vi "HEWH Build Heating Source Array SUo.vi"(4 "Take Sample at 5 Min":bool, 6 "Qr (T), SU0 (F)":bool, 7 "5 Minute Subset Index Adder":i32, 8 "error in (no error)":errorcluster, 9 "Elapsed Time (sec)":dbl[](array[numeric]), 10 "TC Tree Average":dbl[](array[numeric]), 11 "UEF Calculated Values":T1 {"Data Indexes"."15 sec after Draw Index" format="%#.2f"; "Data Indexes"."15 sec after Draw Timestamp" format="%#.2f"; "Data Indexes"."Test Start Timestamp" format="%.2f"; "Data Indexes"."Test End Timestamp" format="%.2f"; "Data Indexes"."T0 Timestamp" format="%.2f"; "Data Indexes"."Tsf Timestamp" format="%.2f"; "Data Indexes"."Tsu0 Timestamp" format="%.2f"; "Data Indexes"."Tmax1 Timestamp" format="%.2f"; "Data Indexes"."Draw Index Timestamp" format="%#.2f"; "Data Indexes"."Non-Draw Timestamp" format="%#.2f"; "Data Indexes"."Heating Timestamp" format="%#.2f"; "Data Indexes"."Start Energy (BTU-Gas)" format="%.6f"; "Data Indexes"."Start Watt Hours" format="%.6f"; "Static Data"."V - Volume of Wh (True)" format="%.5f"; "Static Data"."T-Ambinet Nominal (°F)" format="%.5f"; "Static Data"."T-Inlet Setpoint (°F)" format="%.5f"; "Static Data"."T-Wh Setpoint (°F)" format="%.5f"; "Sampled Data"."Qe (Wh)" format="%.5f"; "Sampled Data"."Tau stby2 (hr)" format="%.5f"; "Sampled Data"."Tastby2 (°F)" format="%.5f"; "Sampled Data"."Qf (BTU)" format="%.5f"; "Sampled Data"."Qe (BTU)" format="%.5f"; "Sampled Data"."Tmax1 (°F)" format="%.5f"; "Sampled Data"."T0 (°F)" format="%.5f"; "Sampled Data"."Qr (BTU)" format="%.5f"; "Sampled Data"."T 24(°F)" format="%.5f"; "Sampled Data"."T astby(°F)" format="%.5f"; "Sampled Data"."T tstby(°F)" format="%.5f"; "Sampled Data"."T su0(°F)" format="%.5f"; "Sampled Data"."T suf(°F)" format="%.5f"; "Sampled Data"."Tau stby_1 (hr)" format="%.5f"; "Sampled Data"."Qsuf (BTU)" format="%.5f"; "Sampled Data"."Qsu0 (BTU)" format="%.5f"; "Calculated Values"."Draw Bonus Volume (gal)" format="%.6f"; "Calculated Values"."Adjustment Factor" format="%.6f"; "Calculated Values"."T*avg_del(n-1)" format="%.6f"; "Calculated Values"."T*min(n-1)" format="%.6f"; "Calculated Values"."T*avg_del(n)" format="%.6f"; "Calculated Values"."Vn" format="%.6f"; "Calculated Values"."Qdm (BTU)" format="%.6f"; "Calculated Values"."QHWD (BTU)" format="%.6f"; "Calculated Values"."QHW (BTU)" format="%.6f"; "Calculated Values"."UEF" format="%.6f"; "Calculated Values"."QHW67 (BTU)" format="%.6f"; "Calculated Values"."Qda (BTU)" format="%.6f"; "Calculated Values"."Qd (BTU)" format="%.6f"; "Calculated Values"."Q (BTU)" format="%.6f"; "Calculated Values"."UA (BTU/(hr*F))" format="%.6f"; "Calculated Values"."Qhr (BTU/hr)" format="%.6f"; "Calculated Values"."Qstby (BTU)" format="%.6f"; "Calculated Values"."nu_r" format="%.6f"; "Calculated Values"."CpUEF (BTU/(lb*F))" format="%.6f"; "Calculated Values"."rho_nu (lb/gal)" format="%.6f"; "Calculated Values"."V1- Vol (Gal)" format="%.6f"; "Calculated Values"."M cluster mass removed (lb)" format="%.6f"; "Calculated Values"."Cp theoretical (BTU/(lbm °F))" format="%.6f"; "Calculated Values"."Tin1 - Mean Inlet 1st Cluster (°F)" format="%.6f"; "Calculated Values"."Tdel1-Mean Outlet 1st Cluster(°F)" format="%.6f"; "Calculated Values"."Cp 24 (BTU/(lb*F))" format="%.6f"; "Calculated Values"."Cp standby (BTU/(lb*F))" format="%.6f"; "Calculated Values"."Cp2 (BTU/(lb*F))" format="%.6f"; "Calculated Values"."Cp1 (BTU/(lb*F))" format="%.6f"; "Calculated Values"."rho 24 (lb/gal)" format="%.6f"; "Calculated Values"."rho standby (lb/gal)" format="%.6f"; "Calculated Values"."rho 2 (lb/gal)" format="%.6f"; "Calculated Values"."Density of cold water All (lbm/gal)" format="%#.3g"; "Calculated Values"."CpHW (BTU/(lbm °F))" format="%#.3g"; "Calculated Values"."Density of hot water All (lbm/gal)" format="%#.3g"; "Calculated Values"."Mass of water All (lbm)" format="%#.3f"}) -> (0 "error out":errorcluster, 1 "Subset Index":i32, 2 "max index(es)":i32, 3 "max value":dbl, 5 "New End Index":i32)   [LabVIEW 2023]
uses:
  Type Definitions/UEF Constants.ctl
  Type Definitions/HEWH Draw Stats.ctl
  Type Definitions/HEWH FHR Draw Type.ctl
  Type Definitions/FHR Bins.ctl
  Type Definitions/HEWH Meter Type.ctl
panel:
  out "subarray":dbl[](array[numeric])
  # "FHR"
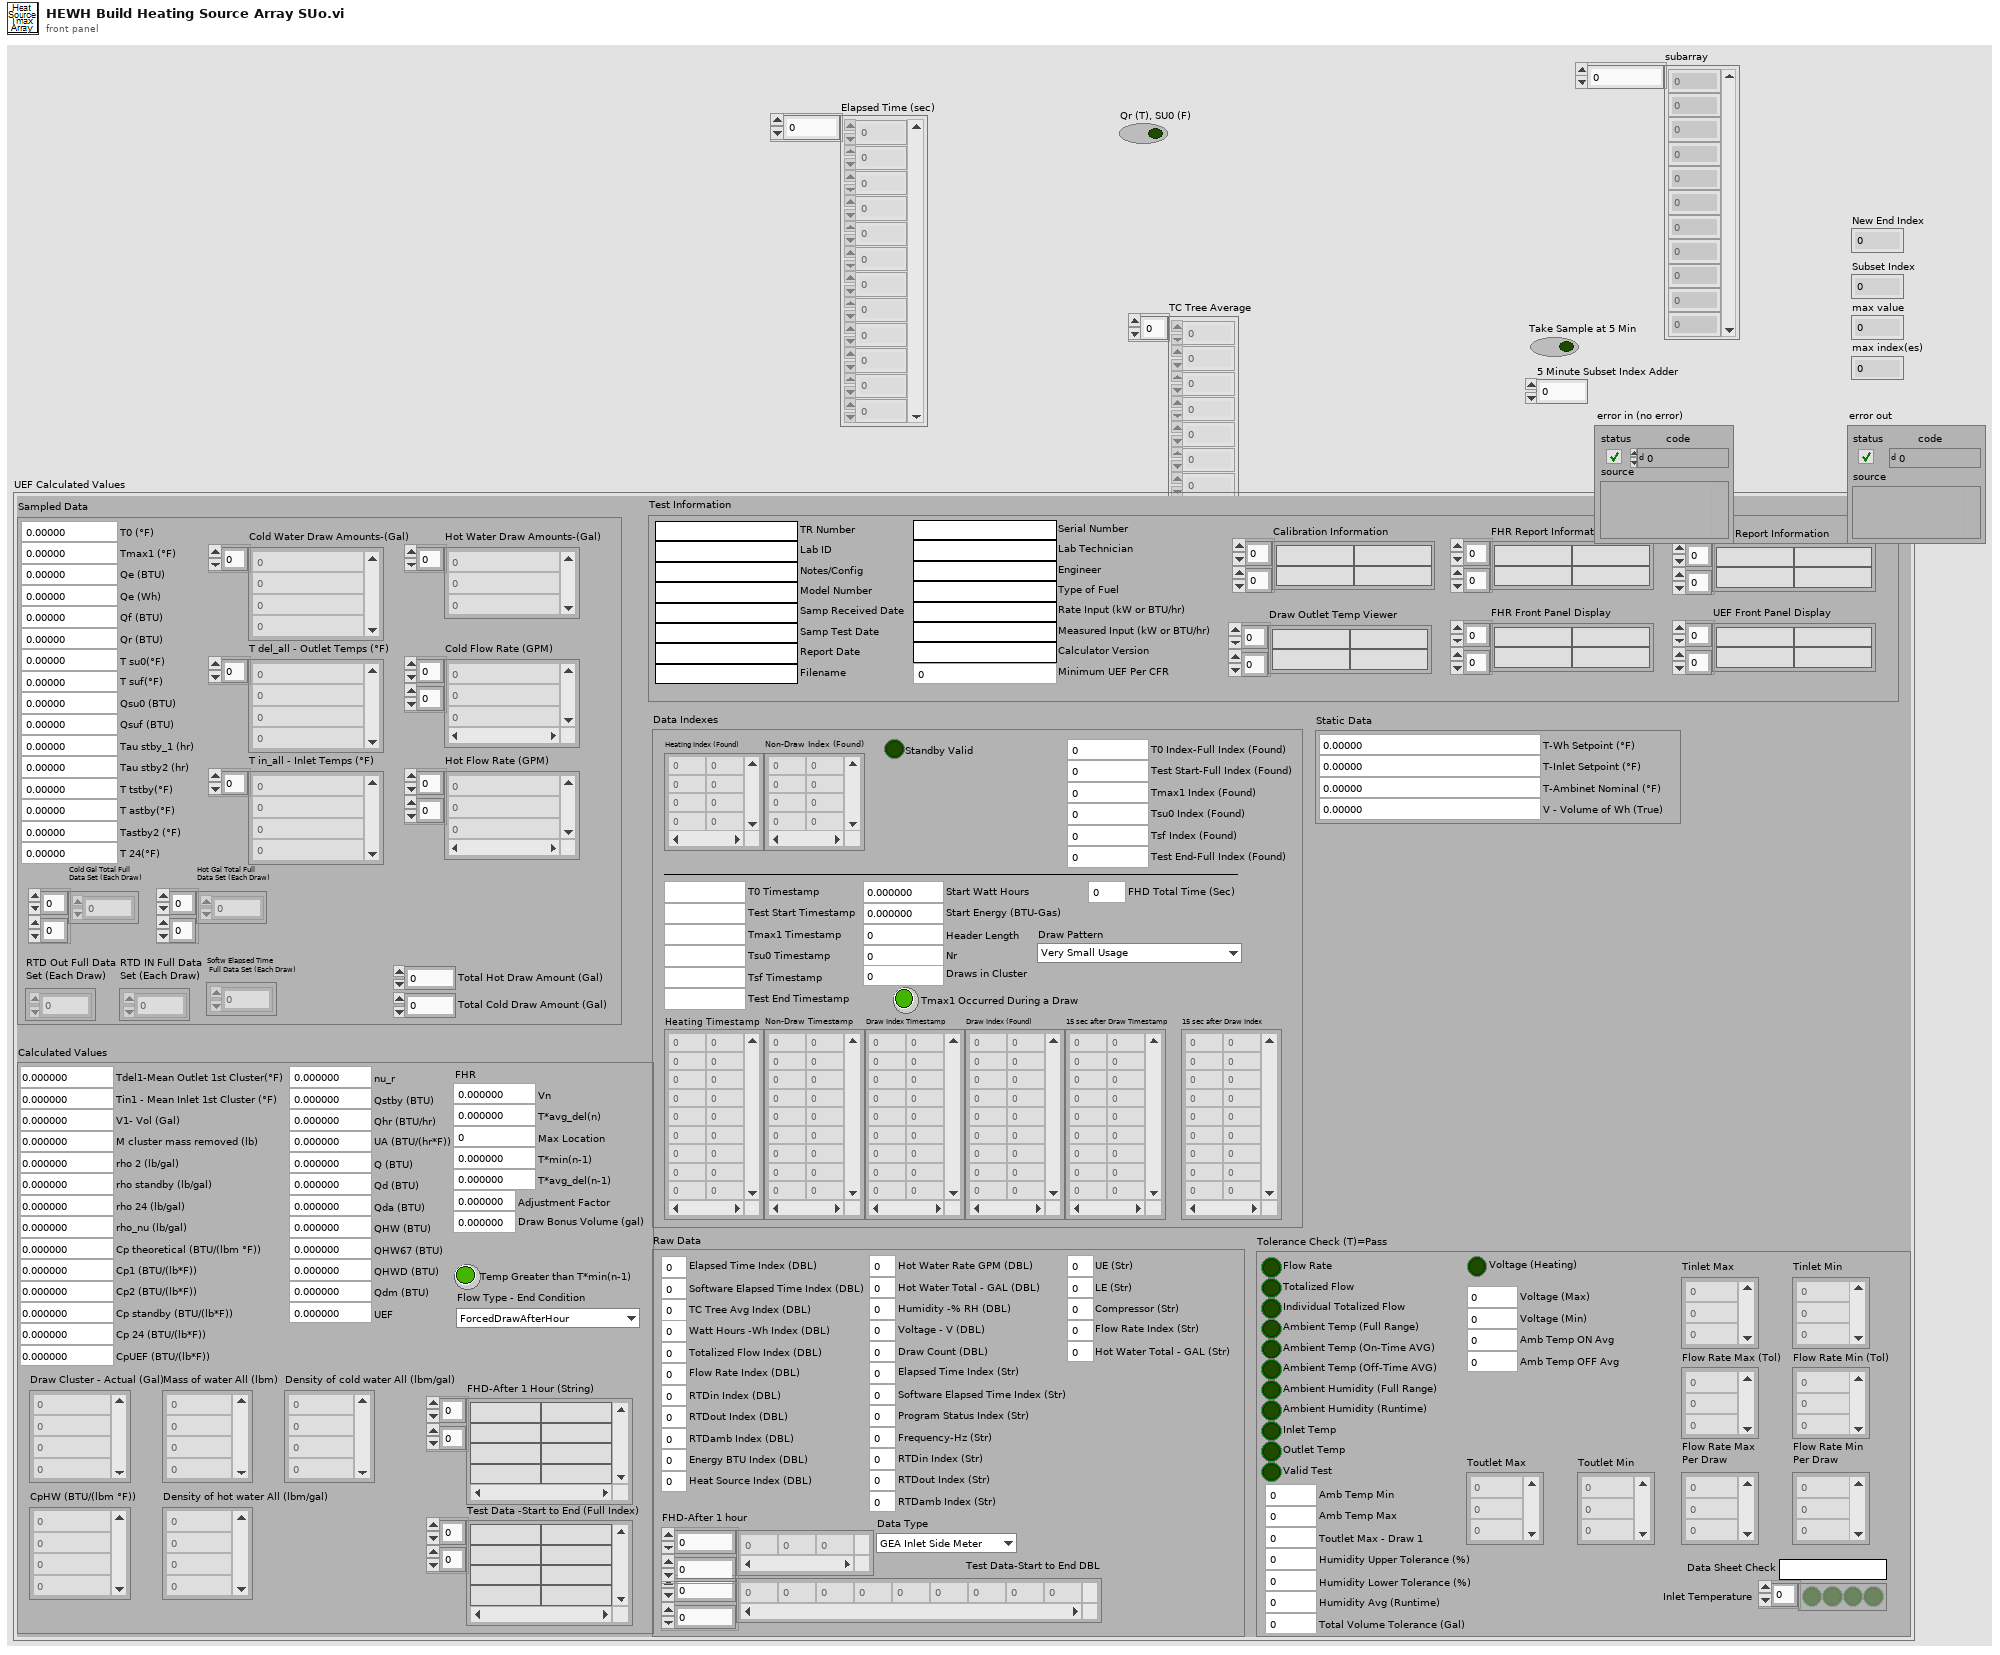
[diagram p1: front panel]
types:
  T1 = typedef "UEF Constants.ctl" = cluster{"Calculated Values":T2, "Sampled Data":cluster{"Cold Water Draw Amounts-(Gal)":dbl[], "T del_all - Outlet Temps (°F)":dbl[], "T in_all - Inlet Temps (°F)":dbl[], "Qsu0 (BTU)":dbl, "Qsuf (BTU)":dbl, "Tau stby_1 (hr)":dbl, "T suf(°F)":dbl, "T su0(°F)":dbl, "T tstby(°F)":dbl, "T astby(°F)":dbl, "T 24(°F)":dbl, "Qr (BTU)":dbl, "T0 (°F)":dbl, "Tmax1 (°F)":dbl, "Qe (BTU)":dbl, "Qf (BTU)":dbl, "Tastby2 (°F)":dbl, "RTD Out Full Data\nSet (Each Draw)":dbl[][], "RTD IN Full Data\nSet (Each Draw)":dbl[][], "Tau stby2 (hr)":dbl, "Hot Water Draw Amounts-(Gal)":dbl[], "Cold Flow Rate (GPM)":dbl[][], "Hot Flow Rate (GPM)":dbl[][], "Softw Elapsed Time\n Full Data Set (Each Draw)":dbl[][], "Cold Gal Total Full\nData Set (Each Draw)":dbl[][], "Total Hot Draw Amount (Gal) ":dbl, "Total Cold Draw Amount (Gal)":dbl, "Qe (Wh)":dbl, "Hot Gal Total Full\nData Set (Each Draw)":dbl[][]}, "Static Data":cluster{"T-Wh Setpoint (°F)":dbl, "T-Inlet Setpoint (°F)":dbl, "T-Ambinet Nominal (°F)":dbl, "V - Volume of Wh (True)":dbl}, "Data Indexes":cluster{"Test Start-Full Index (Found)":i32, "Header Length":i32, "Draw Index (Found)":i32[][], "Nr":i32, "Start Watt Hours":dbl, "Tsu0 Index (Found)":i32, "Tsf Index (Found)":i32, "Start Energy (BTU-Gas)":dbl, "Draws in Cluster":i32, "T0 Index-Full Index (Found)":i32, "Non-Draw Index (Found)":i32[][], "Tmax1 Index (Found)":i32, "Test End-Full Index (Found)":i32, "Heating Index (Found)":i32[][], "Heating Timestamp":dbl[][], "Non-Draw Timestamp":dbl[][], "Draw Index Timestamp":dbl[][], "Tmax1 Timestamp":dbl, "Tsu0 Timestamp":dbl, "Tsf Timestamp":dbl, "T0 Timestamp":dbl, "Test End Timestamp":dbl, "Test Start Timestamp":dbl, "15 sec after Draw Timestamp":dbl[][], "15 sec after Draw Index":dbl[][], "Tmax1 Occurred During a Draw":bool, "FHD Total Time (Sec)":dbl, "Draw Pattern":T4, "Standby Valid":bool}, "Raw Data":cluster{"Elapsed Time Index (DBL)":i32, "Software Elapsed Time Index (DBL)":i32, "TC Tree Avg Index (DBL)":i32, "Watt Hours -Wh Index (DBL)":i32, "Energy BTU Index (DBL)":i32, "Totalized Flow Index (DBL)":i32, "Flow Rate Index (DBL)":i32, "Program Status Index (Str)":i32, "RTDin Index (DBL)":i32, "RTDout Index (DBL)":i32, "RTDamb Index (DBL)":i32, "Test Data-Start to End DBL":dbl[][], "Data Type":T5, "Heat Source Index (DBL)":i32, "Hot Water Rate GPM (DBL)":i32, "Hot Water Total - GAL (DBL)":i32, "FHD-After 1 hour":dbl[][], "Humidity -% RH (DBL)":i32, "Voltage - V (DBL)":i32, "Draw Count (DBL)":i32, "Elapsed Time Index (Str)":i32, "Software Elapsed Time Index (Str)":i32, "Frequency-Hz (Str)":i32, "RTDin Index (Str)":i32, "RTDout Index (Str)":i32, "RTDamb Index (Str)":i32, "UE (Str)":i32, "LE (Str)":i32, "Compressor (Str)":i32, "Flow Rate Index (Str)":i32, "Hot Water Total - GAL (Str)":i32}, "Tolerance Check (T)=Pass":cluster{"Flow Rate":bool, "Totalized Flow":bool, "Ambient Temp (Full Range)":bool, "Ambient Humidity (Full Range)":bool, "Inlet Temp":bool, "Outlet Temp":bool, "Valid Test":bool, "Individual Totalized Flow":bool, "Data Sheet Check":string, "Inlet Temperature":bool[], "Tinlet Max":dbl[], "Tinlet Min":dbl[], "Flow Rate Max (Tol)":dbl[], "Flow Rate Min (Tol)":dbl[], "Amb Temp Max":dbl, "Amb Temp Min":dbl, "Toutlet Max - Draw 1":dbl, "Humidity Upper Tolerance (%)":dbl, "Total Volume Tolerance (Gal)":dbl, "Humidity Lower Tolerance (%)":dbl, "Flow Rate Max\nPer Draw":dbl[], "Flow Rate Min\nPer Draw":dbl[], "Ambient Humidity (Runtime)":bool, "Humidity Avg (Runtime)":dbl, "Ambient Temp (On-Time AVG)":bool, "Ambient Temp (Off-Time AVG)":bool, "Amb Temp OFF Avg":dbl, "Amb Temp ON Avg":dbl, "Voltage (Heating)":bool, "Voltage (Min)":dbl, "Voltage (Max)":dbl, "Toutlet Max":dbl[], "Toutlet Min":dbl[]}, "Test Information":cluster{"TR Number":string, "Lab ID":string, "Notes/Config":string, "Model Number":string, "Serial Number":string, "Lab Technician":string, "Engineer":string, "Type of Fuel":string, "Samp Received Date":string, "Samp Test Date":string, "Report Date":string, "Rate Input (kW or BTU/hr)":string, "Measured Input (kW or BTU/hr)":string, "Filename":string, "Calibration Information":string[][], "Calculator Version":string, "Minimum UEF Per CFR":dbl, "UEF Report Information":string[][], "FHR Report Information":string[][], "FHR Front Panel Display":string[][], "UEF Front Panel Display":string[][], "Draw Outlet Temp Viewer":string[][]}}
  T2 = typedef "HEWH Draw Stats.ctl" = cluster{"Draw Cluster - Actual (Gal)":dbl[], "Mass of water All (lbm)":dbl[], "Density of hot water All (lbm/gal)":dbl[], "CpHW (BTU/(lbm °F))":dbl[], "rho 2 (lb/gal)":dbl, "rho standby (lb/gal)":dbl, "rho 24 (lb/gal)":dbl, "Cp1 (BTU/(lb*F))":dbl, "Cp2 (BTU/(lb*F))":dbl, "Cp standby (BTU/(lb*F))":dbl, "Cp 24 (BTU/(lb*F))":dbl, "nu_r":dbl, "Qstby (BTU)":dbl, "Qhr (BTU/hr)":dbl, "UA (BTU/(hr*F))":dbl, "Q (BTU)":dbl, "Qd (BTU)":dbl, "Qda (BTU)":dbl, "QHW67 (BTU)":dbl, "UEF":dbl, "Tdel1-Mean Outlet 1st Cluster(°F)":dbl, "Tin1 - Mean Inlet 1st Cluster (°F)":dbl, "Cp theoretical (BTU/(lbm °F))":dbl, "M cluster mass removed (lb)":dbl, "V1- Vol (Gal)":dbl, "Test Data -Start to End (Full Index)":string[][], "rho_nu (lb/gal)":dbl, "Density of cold water All (lbm/gal)":dbl[], "CpUEF (BTU/(lb*F))":dbl, "QHW (BTU)":dbl, "QHWD (BTU)":dbl, "Qdm (BTU)":dbl, "FHD-After 1 Hour (String)":string[][], "Vn":dbl, "T*avg_del(n)":dbl, "Max Location":i32, "T*min(n-1)":dbl, "T*avg_del(n-1)":dbl, "Temp Greater than T*min(n-1)":bool, "Adjustment Factor":dbl, "Draw Bonus Volume (gal)":dbl, "Flow Type - End Condition":T3}
  T3 = typedef "HEWH FHR Draw Type.ctl" = enum16{"ForcedDrawAfterHour", "HeatingCutoffBeforeHour"}
  T4 = typedef "FHR Bins.ctl" = enum16{"Very Small Usage", "Low Usage", "Medium Usage", "High Usage", "Undefined"}
  T5 = typedef "HEWH Meter Type.ctl" = enum16{"GEA Inlet Side Meter", "GEA Outlet Side Meter", "CSA Inlet Side Meter"}
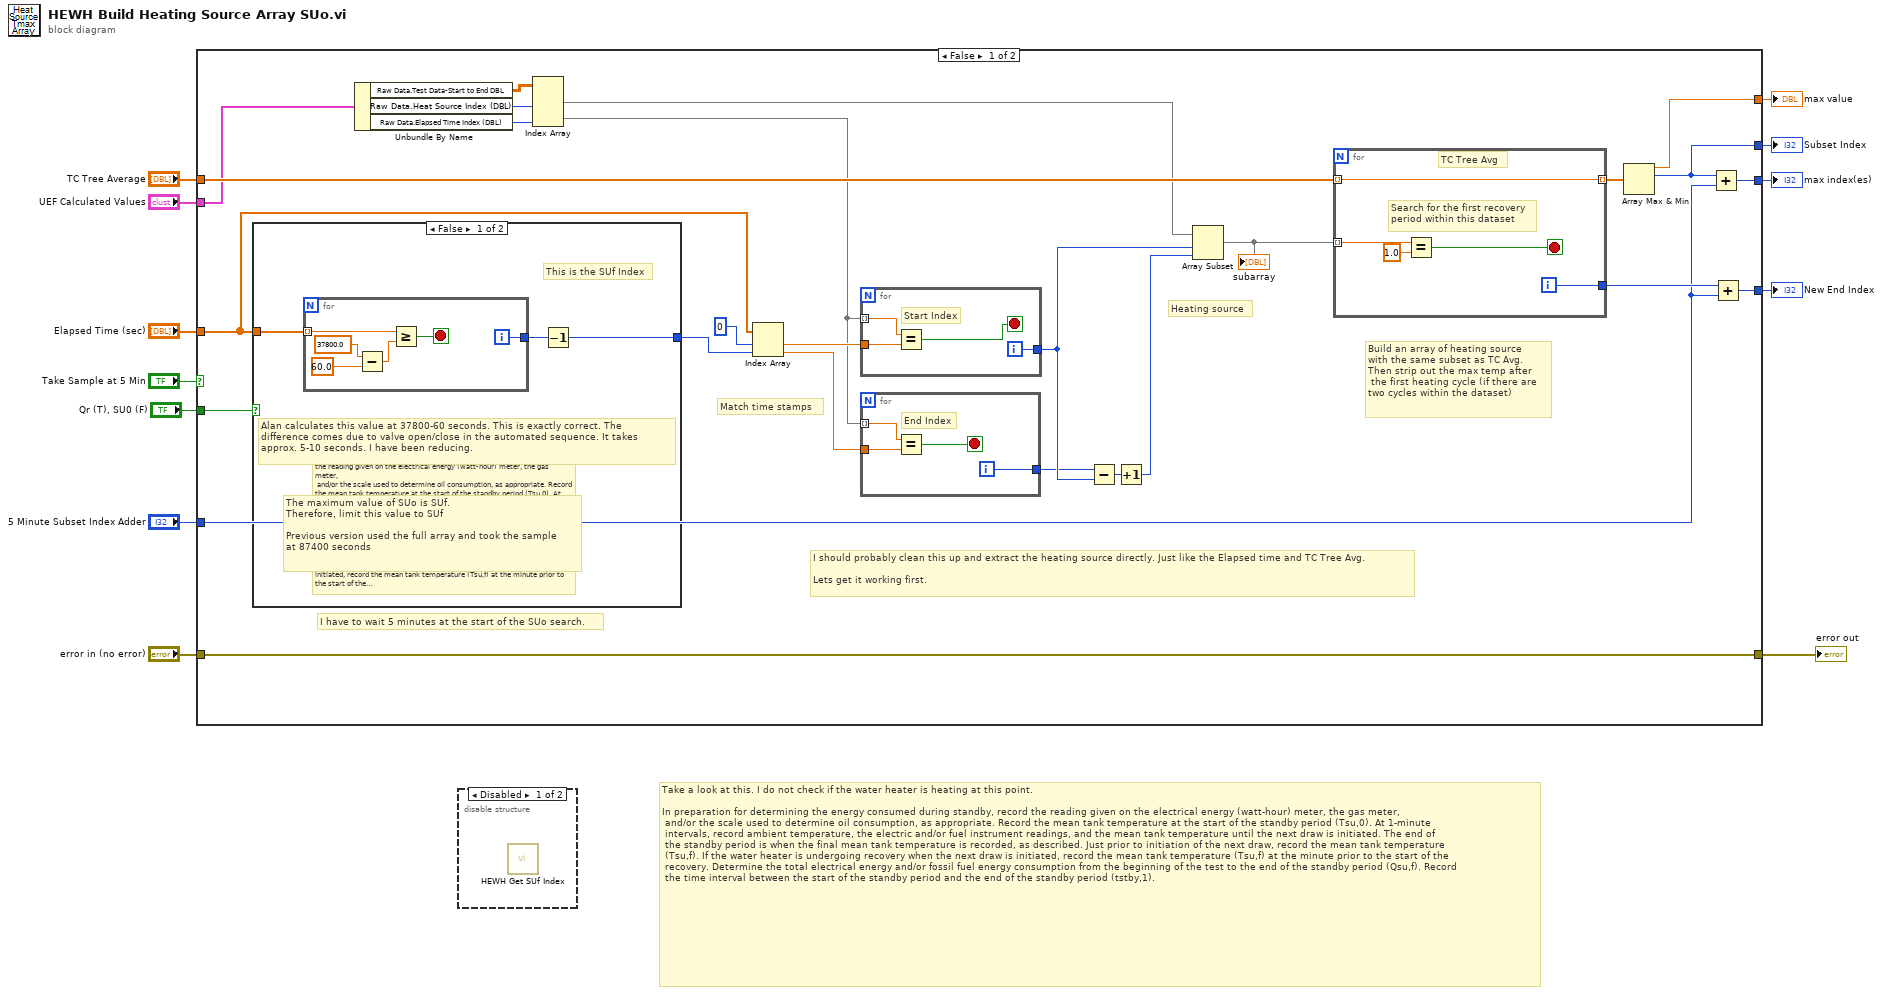
[diagram p0: block diagram]
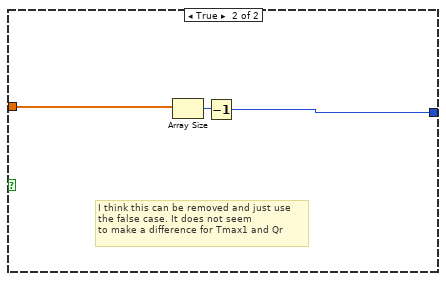
[diagram p3: hidden frame]
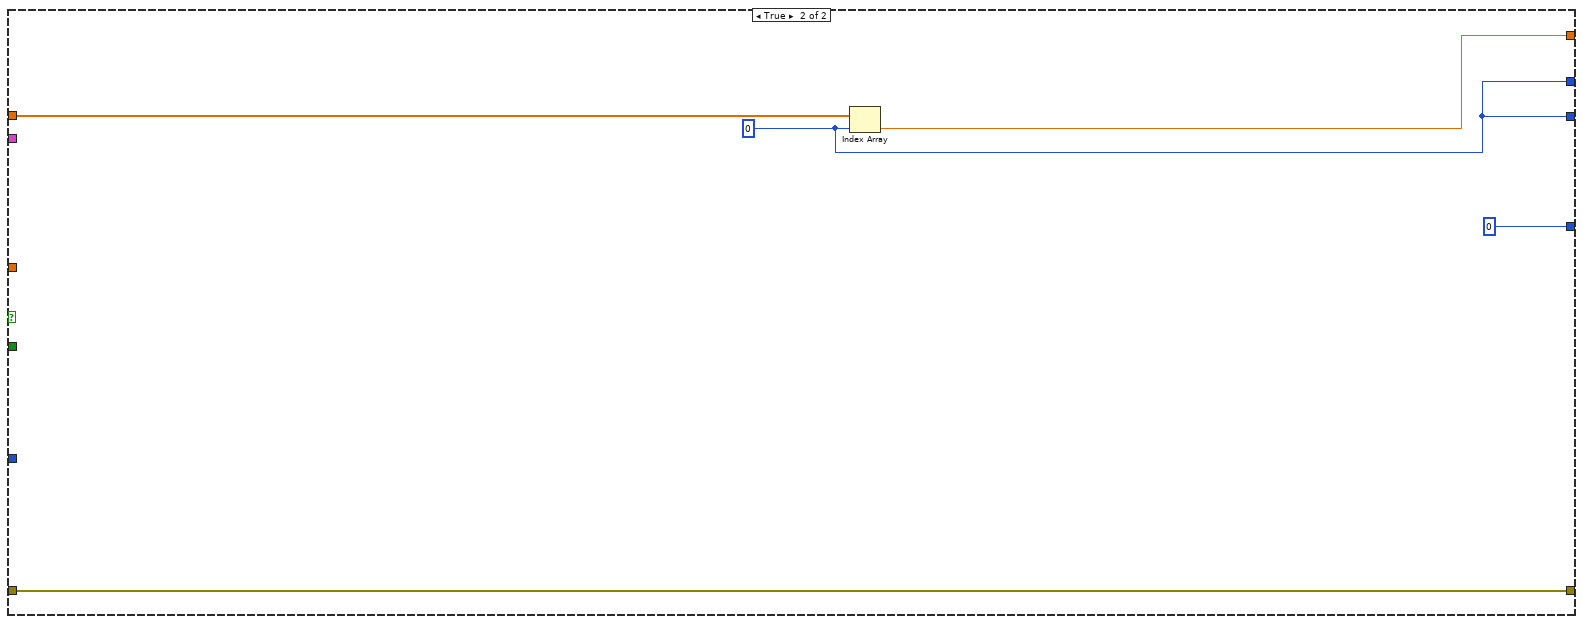
[diagram p4: hidden frame]
diagram:
  # "Take a look at this. I do not check if the water heater is heating at this point. \n\nIn preparation for determining the energy consumed during standby, record the reading given on the electrical energy (watt-hour) meter, the gas meter,\n and/or the scale used to determine oil consumption, as appropriate. Record the mean tank temperature at the start of the standby period (Tsu,0). At 1-minute\n intervals, record ambient temperature, the electric and/or fuel instrument readings, and the mean tank temperature until the next draw is initiated. The end of\n the standby period is when the final mean tank temperature is recorded, as described. Just prior to initiation of the next draw, record the mean tank temperature\n (Tsu,f). If the water heater is undergoing recovery when the next draw is initiated, record the mean tank temperature (Tsu,f) at the minute prior to the start of the\n recovery. Determine the total electrical energy and/or fossil fuel energy consumption from the beginning of the test to the end of the standby period (Qsu,f). Record\n the time interval between the start of the standby period and the end of the standby period (tstby,1)."
  n1 = case shown="False" "Take Sample at 5 Min" {
    tunnel: "TC Tree Average" -> [w38 w68]
    tunnel: "Elapsed Time (sec)" -> [w13 _]
    tunnel: [w37 w66] -> w10
    tunnel: "UEF Calculated Values" -> [w26 _]
    tunnel: [w25 w65] -> w8
    tunnel: "5 Minute Subset Index Adder" -> [w21 _]
    tunnel: [w24 w65] -> w6
    tunnel: [w23 w67] -> w5
    tunnel: "error in (no error)" -> [w23 w67]
    tunnel: [w20 0] -> w2
    tunnel: "Qr (T), SU0 (F)" -> [w18 _]
    frame False {
      # "I have to wait 5 minutes at the start of the SUo search."
      # "I should probably clean this up and extract the heating source directly. Just like the Elapsed time and TC Tree Avg. \n\nLets get it working first."
      # "Build an array of heating source\nwith the same subset as TC Avg.\nThen strip out the max temp after\n the first heating cycle (if there are \ntwo cycles within the dataset)"
      # "Match time stamps"
      # "Heating source"
      n2 = case shown="False" w18 {
        tunnel: w13 -> [w39 w48]
        tunnel: [w40 w49] -> w19
        frame False {
          # "This is the SUf Index"
          # "Alan calculates this value at 37800-60 seconds. This is exactly correct. The \ndifference comes due to valve open/close in the automated sequence. It takes \napprox. 5-10 seconds. I have been reducing."
          # "Take a look at this. I do not check if the water heater is heating at this point. \n\nIn preparation for determining the energy consumed during standby, record the reading given on the electrical energy (watt-hour) meter, the gas meter,\n and/or the scale used to determine oil consumption, as appropriate. Record the mean tank temperature at the start of the standby period (Tsu,0). At 1-minute\n intervals, record ambient temperature, the electric and/or fuel instrument readings, and the mean tank temperature until the next draw is initiated. The end of\n the standby period is when the final mean tank temperature is recorded, as described. Just prior to initiation of the next draw, record the mean tank temperature\n (Tsu,f). If the water heater is undergoing recovery when the next draw is initiated, record the mean tank temperature (Tsu,f) at the minute prior to the start of the\n recovery. Determine the total electrical energy and/or fossil fuel energy consumption from the beginning of the test to the end of the standby period (Qsu,f). Record\n the time interval between the start of the standby period and the end of the standby period (tstby,1)."
          # "The maximum value of SUo is SUf.\nTherefore, limit this value to SUf\n\nPrevious version used the full array and took the sample\nat 87400 seconds"
          n3 = for {
            tunnel: w39 -> [w42] mode=indexing
            tunnel: [w46] -> w41
            i -> [w46]
            stop <- w47 stop-if-true
            n4 = Subtract(x=37800.0 ("y"), y=60.0) -> (x-y=w43:dbl)
            n5 = Greater Or Equal?(x=w42, y=w43) -> (x >= y?=w47:bool)
          }
          n6 = Decrement(x=w41) -> (x-1=w40:i32)
        }
        frame True {
          # "I think this can be removed and just use\nthe false case. It does not seem \nto make a difference for Tmax1 and Qr"
          n7 = Array Size(array=w48) -> (size(s)=w50:i32)
          n8 = Decrement(x=w50) -> (x-1=w49:i32)
        }
      }
      n9 = Unbundle By Name(w26) -> ("Raw Data.Test Data-Start to End DBL"=w27:dbl[][], "Raw Data.Heat Source Index (DBL)"=w17:i32, "Raw Data.Elapsed Time Index (DBL)"=w16:i32)
      n10 = Index Array(array=w27, index (col) #1=w17, index (col) #2=w16) -> (element #1=w15:dbl[], element #2=w14:dbl[])  [unwired: 2 in]
      n11 = Index Array(array=w13, index #1=0 ("index"), index #2=w19) -> (element #1=w29:dbl, element #2=w30:dbl)
      n12 = for {
        tunnel: w14 -> [w63] mode=indexing
        tunnel: w29 -> [w62]
        tunnel: [w60] -> w33
        i -> [w60]
        stop <- w61 stop-if-true
        # "Start Index"
        n13 = Equal?(x=w63, y=w62) -> (x = y?=w61:bool)
      }
      n14 = for {
        tunnel: w14 -> [w59] mode=indexing
        tunnel: w30 -> [w58]
        tunnel: [w56] -> w31
        i -> [w56]
        stop <- w57 stop-if-true
        # "End Index"
        n15 = Equal?(x=w59, y=w58) -> (x = y?=w57:bool)
      }
      n16 = Subtract(x=w31, y=w33) -> (x-y=w32:i32)
      n17 = Increment(x=w32) -> (x+1=w34:i32)
      n18 = Array Subset(array=w15, index=w33, length=w34) -> (w35:dbl[])
      "subarray" <- w35
      n19 = for {
        tunnel: w35 -> [w55] mode=indexing
        tunnel: [w52] -> w36 mode=indexing
        tunnel: w38 -> [w52] mode=indexing
        tunnel: [w51] -> w22
        i -> [w51]
        stop <- w53 stop-if-true
        # "TC Tree Avg"
        # "Search for the first recovery\nperiod within this dataset"
        n20 = Equal?(x=w55, y=1.0) -> (x = y?=w53:bool)
      }
      n21 = Array Max & Min(array=w36) -> (max value=w37:dbl, max index (indices)=w25:i32)  [unwired: 2 out]
      n22 = Add(x=w25, y=w21) -> (x+y=w24:i32)
      n23 = Add(x=w22, y=w21) -> (x+y=w20:i32)
    }
    frame True {
      w65 = 0 ("index")
      n24 = Index Array(array=w68, index=w65) -> (element=w66:dbl)
    }
  }
  "max value" <- w10
  "max index(es)" <- w6
  "error out" <- w5
  "Subset Index" <- w8
  "New End Index" <- w2
  n25 = disable-structure shown="Disabled" {
    frame Disabled {
      n26 = call "HEWH Get SUf Index.vi"() -> ()  [unwired: 10 in, 2 out]
    }
    frame Enabled {
    }
  }
